vi "Get Transform Matrix.vi"(8 "error in (no error)":errorcluster, 9 "Glyph Size":cluster{"Width":sgl, "Height":sgl}, 10 "Canvas Size":cluster{"Width":i32, "Height":i32}, 11 "Static Image Transform in":refnum<class "Static Image Transform.lvclass">) -> (0 "error out":errorcluster, 2 "Transform":T1, 3 "Static Image Transform out":refnum<class "Static Image Transform.lvclass">)   [LabVIEW 2023, in "Glyph Drawer.lvlib" / "Static Image Transform.lvclass"]
uses:
  Static Image Transform.lvclass
  <vilib>/Analysis/Matrix/Datatypes/RealMatrix.ctl
  Static Image Transform.lvclass/Static Image Transform.ctl
  <vilib>/Analysis/baseanly.llb/Real A x B.vi
  Glyph Drawer.lvlib
  <vilib>/Analysis/Matrix/NI_Matrix.lvlib
  <vilib>/Analysis/NI_AALBase.lvlib
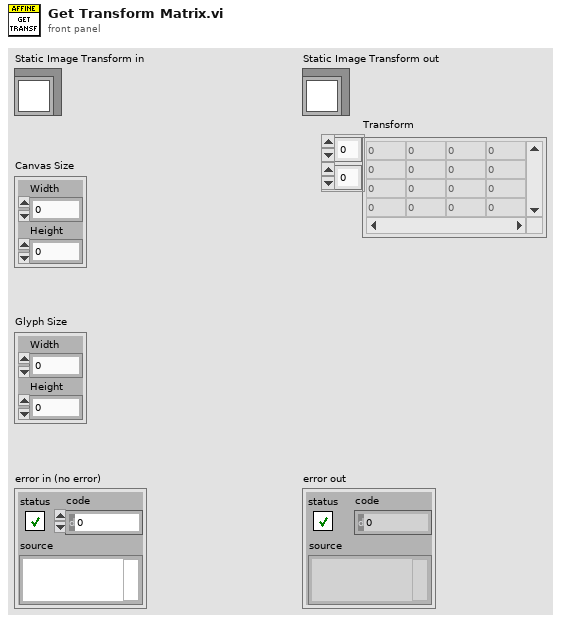
[diagram p1: front panel]
types:
  T1 = typedef "NI_Matrix.lvlib/RealMatrix.ctl" = dbl[][]
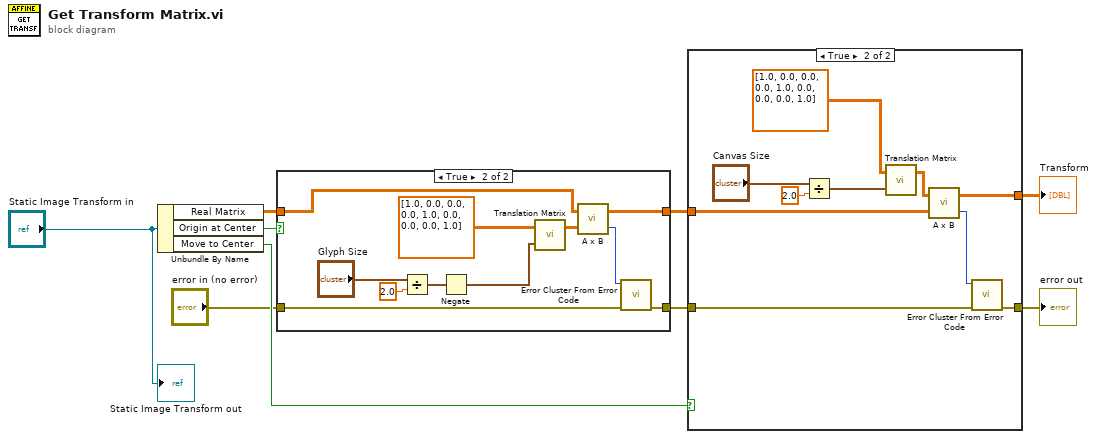
[diagram p0: block diagram]
diagram:
  n1 = Unbundle By Name("Static Image Transform in") -> ("Real Matrix"=w8:T1, "Origin at Center"=w7:bool, "Move to Center"=w6:bool)
  n2 = case shown="True" w7 {
    tunnel: w8 -> [w11 w22]
    tunnel: [w11 w17] -> w1
    tunnel: "error in (no error)" -> [w10 w15]
    tunnel: [w10 w14] -> w3
    frame False {
    }
    frame True {
      n3 = Divide(x="Glyph Size", y=2.0) -> (x/y=w20:cluster{"Width":dbl, "Height":dbl})
      n4 = Negate(x=w20) -> (-x=w12:cluster{"Width":dbl, "Height":dbl})
      n5 = call "Translation Matrix.vi"("Translation"=w12, "Matrix Type (2x3)"=T1 [[1.0, 0.0, 0.0], [0.0, 1.0, 0.0], [0.0, 0.0, 1.0]]) -> ("Matrix Out"=w16:T1)  [unwired: 1 in]
      n6 = call-poly <vilib>:"A x B.vi"("B"=w16, "A"=w22) -> ("error"=w13:i32, "A x B"=w17:T1)
      n7 = call <vilib>:"Error Cluster From Error Code.vi"("error in (no error)"=w15, "error code (0)"=w13) -> ("error out"=w14:errorcluster)  [unwired: 7 in]
    }
  }
  n8 = case shown="True" w6 {
    tunnel: w1 -> [w24 w34]
    tunnel: [w24 w31] -> w5
    tunnel: w3 -> [w23 w28]
    tunnel: [w23 w27] -> w2
    frame False {
    }
    frame True {
      n9 = Divide(x="Canvas Size", y=2.0) -> (x/y=w25:cluster{"Width":dbl, "Height":dbl})
      n10 = call "Translation Matrix.vi"("Translation"=w25, "Matrix Type (2x3)"=T1 [[1.0, 0.0, 0.0], [0.0, 1.0, 0.0], [0.0, 0.0, 1.0]]) -> ("Matrix Out"=w30:T1)  [unwired: 1 in]
      n11 = call-poly <vilib>:"A x B.vi"("B"=w34, "A"=w30) -> ("error"=w26:i32, "A x B"=w31:T1)
      n12 = call <vilib>:"Error Cluster From Error Code.vi"("error in (no error)"=w28, "error code (0)"=w26) -> ("error out"=w27:errorcluster)  [unwired: 7 in]
    }
  }
  "error out" <- w2
  "Transform" <- w5
  "Static Image Transform out" <- "Static Image Transform in"
